vi "Basic FileIO.vi"() -> ()   [LabVIEW 2016]
uses:
  <vilib>/Analysis/2dsp.llb/2D Convolution (DBL).vi
  <vilib>/picture/picture.llb/Draw True-Color Pixmap.vi
  <vilib>/Analysis/NI_AALPro.lvlib
panel:
  out "Enhanced":picture
  out "Src":picture
  out "Reversed":picture
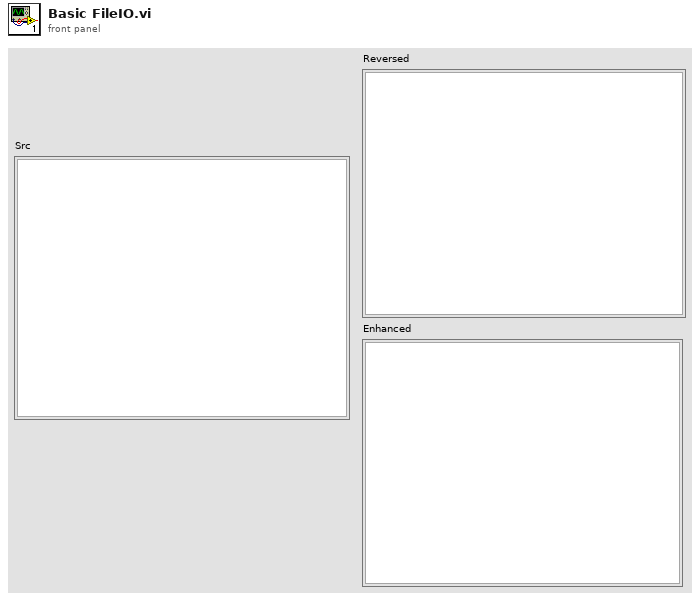
[diagram p1: front panel]
types:
  T1 = typedef "imagedata.ctl" = cluster{"image type":i32, "image depth":i32, "image":u8[], "mask":u8[], "colors":u32[], "Rectangle":cluster{"left":i16, "top":i16, "right":i16, "bottom":i16}}
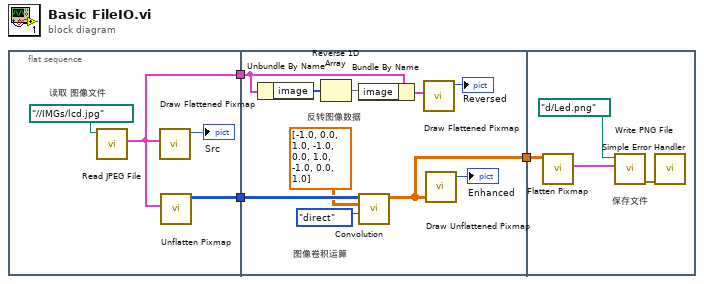
[diagram p0: block diagram]
diagram:
  n1 = flat-sequence {
    tunnel: [w5] -> w3
    tunnel: [w4] -> w2
    tunnel: w3 -> [w13]
    tunnel: w2 -> [w12]
    tunnel: [w8] -> w1
    tunnel: w1 -> [w18]
    frame #0 {
      # "读取 图像文件"
      n2 = call <vilib>:"Read JPEG File.vi"("path to JPEG file"=path "../../IMGs/lcd.jpg" ("path to PNG file")) -> ("image data"=w5:T1)  [unwired: 8 in, 2 out]
      n3 = call <vilib>:"Draw Flattened Pixmap.vi"("image data"=w5) -> ("new picture"=→"Src":picture)  [unwired: 8 in]
      n4 = call <vilib>:"Unflatten Pixmap.vi"("image data"=w5) -> ("24-bit pixmap"=w4:u32[][])  [unwired: 4 in, 6 out]
    }
    frame #1 {
      # "图像卷积运算"
      # "反转图像数据"
      n5 = Unbundle By Name(w13) -> ("image"=w17:u8[])
      n6 = Reverse 1D Array(array=w17) -> (reversed array=w15:u8[])
      n7 = Bundle By Name(cluster=w13, "image"=w15) -> (w16:T1)
      n8 = call-poly <vilib>:"Convolution.vi"("algorithm"=enum32{"direct", "frequency domain"}."direct", "Y"=dbl[][] [[-1.0, 0.0, 1.0], [-1.0, 0.0, 1.0], [-1.0, 0.0, 1.0]], "X"=w12) -> ("X * Y"=w8:dbl[][])  [unwired: 7 in, 1 out]
      n9 = call <vilib>:"Draw Flattened Pixmap.vi"("image data"=w16) -> ("new picture"=→"Reversed":picture)  [unwired: 8 in]
      n10 = call-poly <vilib>:"Draw Unflattened Pixmap.vi"("data (RGB format)"=w8) -> ("new picture"=→"Enhanced":picture)  [unwired: 8 in]
    }
    frame #2 {
      # "保存文件"
      n11 = call <vilib>:"Flatten Pixmap.vi"("24-bit pixmap"=w18) -> ("image data"=w21:T1)  [unwired: 10 in]
      n12 = call <vilib>:"Write PNG File.vi"("image data"=w21, "path to PNG file"=path "d:/Led.png") -> ("error out"=w19:errorcluster)  [unwired: 8 in, 1 out]
      n13 = call <vilib>:"Simple Error Handler.vi"("error in (no error)"=w19) -> ()  [unwired: 4 in, 5 out]
    }
  }
